vi "take_image_sbig.vi"(1 "Exptime":dbl, 2 "path":path) -> (0 "error out":errorcluster)   [LabVIEW 2020]
panel:
  out "appended path":path
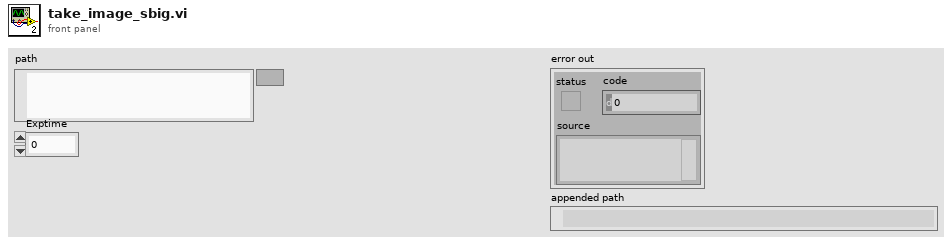
[diagram p1: front panel]
types:
  T1 = enum16{"open", "replace", "create", "open or create", "replace or create", "replace or create with confirmation"}
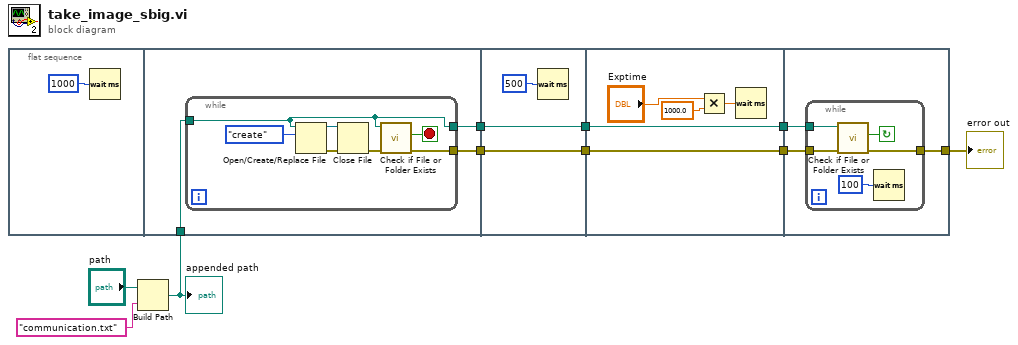
[diagram p0: block diagram]
diagram:
  n1 = flat-sequence {
    tunnel: w8 -> [w14]
    tunnel: [w13] -> w7
    tunnel: [w12] -> w6
    tunnel: [w23] -> w4
    tunnel: w7 -> [w23]
    tunnel: [w22] -> w3
    tunnel: w6 -> [w22]
    tunnel: [w26] -> w2
    tunnel: w4 -> [w26]
    tunnel: [w25] -> w1
    tunnel: w3 -> [w25]
    tunnel: w2 -> [w32]
    tunnel: w1 -> [w31]
    tunnel: [w30] -> w5
    frame #0 {
      n2 = Wait (ms)(milliseconds to wait=u32 1000) -> ()  [unwired: 1 out]
    }
    frame #1 {
      n3 = while {
        tunnel: w14 -> [w18]
        tunnel: [w18] -> w13
        tunnel: [w20] -> w12
        stop <- w21 stop-if-true
        n4 = Open/Create/Replace File(file path (use dialog)=w18, operation (0:open)=T1."create") -> (refnum out=w19:refnum<file>, error out=w17:errorcluster)  [unwired: 4 in, 1 out]
        n5 = Close File(refnum=w19, error in=w17) -> (error out=w16:errorcluster)  [unwired: 1 out]
        n6 = call <vilib>:"Check if File or Folder Exists.vi"("error in (no error)"=w16, "path"=w18) -> ("error out"=w20:errorcluster, "file or folder exists?"=w21:bool)  [unwired: 7 in, 1 out]
      }
    }
    frame #2 {
      n7 = Wait (ms)(milliseconds to wait=u32 500) -> ()  [unwired: 1 out]
    }
    frame #3 {
      n8 = Multiply(x="Exptime", y=1000.0) -> (x*y=w28:dbl)
      n9 = Wait (ms)(milliseconds to wait=w28) -> ()  [unwired: 1 out]
    }
    frame #4 {
      n10 = while {
        tunnel: w32 -> [w35]
        tunnel: w31 -> [w34]
        tunnel: [w33] -> w30
        stop <- w37 continue-if-true
        n11 = call <vilib>:"Check if File or Folder Exists.vi"("error in (no error)"=w34, "path"=w35) -> ("error out"=w33:errorcluster, "file or folder exists?"=w37:bool)  [unwired: 7 in, 1 out]
        n12 = Wait (ms)(milliseconds to wait=u32 100) -> ()  [unwired: 1 out]
      }
    }
  }
  n13 = Build Path(base path="path", name or relative path="communication.txt") -> (appended path=w8:path)
  "appended path" <- w8
  "error out" <- w5
